vi "Set BufferLastReadsDBL.vi"(10 "BufferLastReadsDBL.lvclass":refnum<class "BufferLastReadsDBL.lvclass">, 11 "DAQmx BufferLastReadsDBL in":refnum<class "DAQmx BufferLastReadsDBL.lvclass">) -> (3 "DAQmx BufferLastReadsDBL out":refnum<class "DAQmx BufferLastReadsDBL.lvclass">)   [LabVIEW 2024, in "DAQmx BufferLastReadsDBL.lvclass"]
uses:
  DAQmx BufferLastReadsDBL.lvclass
  Buffers/BufferLastReadingsDBL/BufferLastReadsDBL.lvclass
  DAQmx BufferLastReadsDBL.lvclass/DAQmx BufferLastReadsDBL.ctl
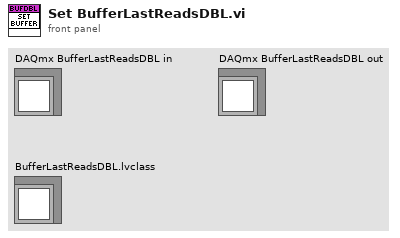
[diagram p1: front panel]
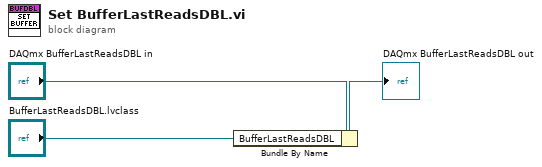
[diagram p0: block diagram]
diagram:
  n1 = Bundle By Name(cluster="DAQmx BufferLastReadsDBL in", "BufferLastReadsDBL"="BufferLastReadsDBL.lvclass") -> (→"DAQmx BufferLastReadsDBL out":refnum<class "DAQmx BufferLastReadsDBL.lvclass">)
